vi "Destroy.vi"(0 "reference in":refnum<class "TEXT.lvclass">, 5 "error in (no error)":errorcluster) -> (14 "reference out":refnum<class "TEXT.lvclass">, 19 "error out":errorcluster)   [LabVIEW 2020, in "TEXT.lvclass"]
doc: "Destructor."
uses:
  TEXT.lvclass
  API/Generic Utilities_class/Generic Utilities.lvclass
  API/GSwFormDSP_class/GSwFormDSP.lvclass
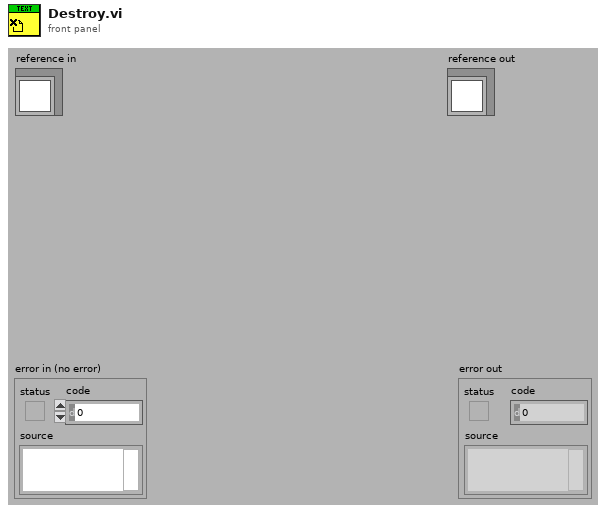
[diagram p1: front panel]
types:
  T1 = typedef "TEXT.lvclass/ObjectAttributes.ctl" = cluster{"Time Data":refnum<class "GSwFormDSP.lvclass">, "New Time Data Obj?":bool}
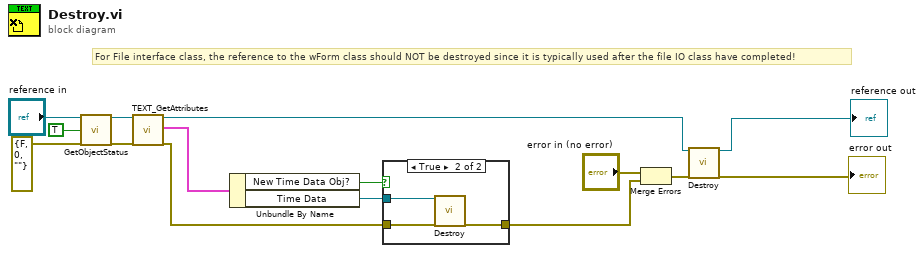
[diagram p0: block diagram]
diagram:
  # "For File interface class, the reference to the wForm class should NOT be destroyed since it is typically used after the file IO class have completed!"
  n1 = call-dynamic "GetObjectStatus.vi"("reference in"="reference in", "simple info (F)"=TRUE ("simple info"), "error in (no error)"=errorcluster {"status"=FALSE, "code"=0, "source"=""}) -> ("reference out"=w6:refnum<class "TEXT.lvclass">, "error out"=w4:errorcluster)  [unwired: 5 in, 10 out]
  n2 = call "TEXT_GetAttributes.vi"("reference in"=w6, "error in (no error)"=w4) -> ("reference out"=w5:refnum<class "TEXT.lvclass">, "attributes"=w2:T1, "error out"=w3:errorcluster)  [unwired: 14 in, 1 out]
  n3 = Unbundle By Name(w2) -> ("New Time Data Obj?"=w7:bool, "Time Data"=w8:refnum<class "GSwFormDSP.lvclass">)
  n4 = case shown="True" w7 {
    tunnel: w8 -> [_ w19]
    tunnel: w3 -> [w16 w18]
    tunnel: [w16 w17] -> w1
    frame False {
    }
    frame True {
      n5 = call-dynamic "Destroy.vi"("reference in"=w19, "error in (no error)"=w18) -> ("error out"=w17:errorcluster)  [unwired: 16 in, 1 out]
    }
  }
  n6 = Merge Errors("error in (no error)", w1) -> (w14:errorcluster)
  n7 = call-parent "Destroy.vi"("reference in"=w5, "error in (no error)"=w14) -> ("reference out"=→"reference out":refnum<class "TEXT.lvclass">, "error out"=→"error out":errorcluster)  [unwired: 16 in]
